vi "Get Short Help.vi"(8 "error in (no error)":errorcluster, 11 "Install in":refnum<class "Install.lvclass">) -> (0 "error out":errorcluster, 2 "Short Help":string, 3 "Install out":refnum<class "Install.lvclass">)   [LabVIEW 2020, in "Install.lvlib" / "Install.lvclass"]
uses:
  Install.lvclass
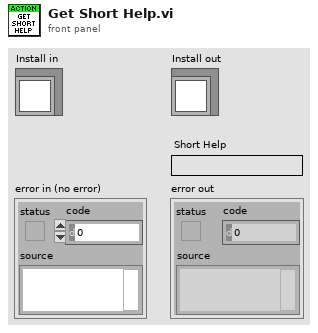
[diagram p1: front panel]
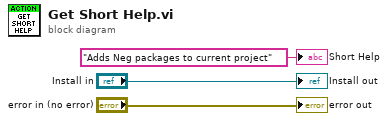
[diagram p0: block diagram]
diagram:
  "error out" <- "error in (no error)"
  "Install out" <- "Install in"
  "Short Help" <- "Adds Neg packages to current project" ("Short Help")
